vi "Euler sieve.vi"() -> ()   [LabVIEW 2021]
uses:
  <vilib>/Utility/file.llb/Write Delimited Spreadsheet (I64).vi
panel:
  in  "Path":path
  out "Running Time":dbl
  out "Array 2":u64[](array[numeric])
  out "Array":bool[](array[boolean])
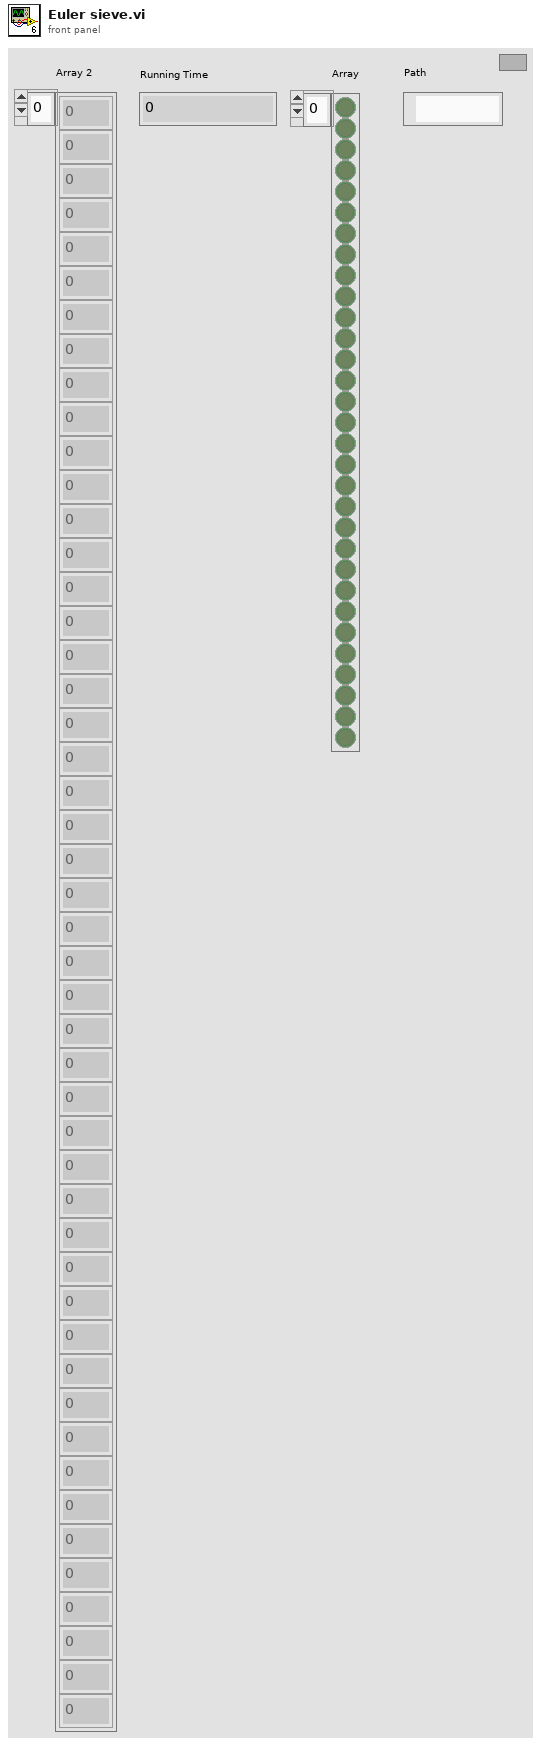
[diagram p1: front panel]
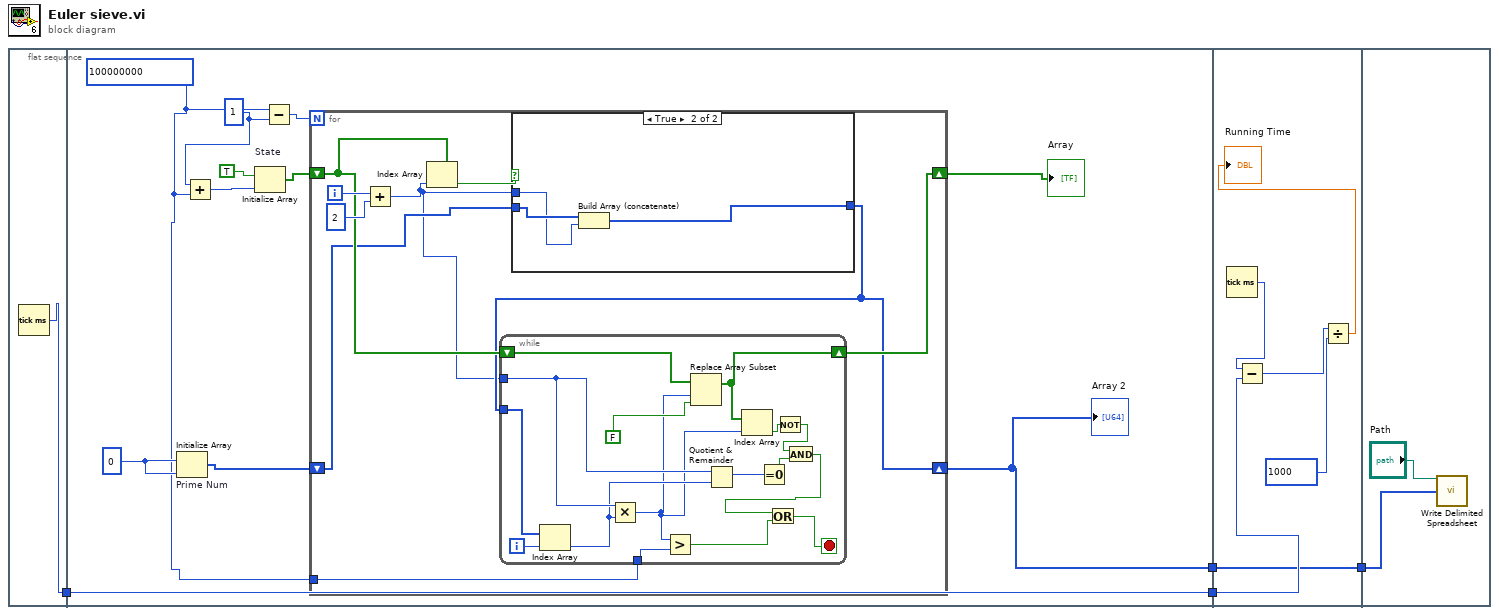
[diagram p0: block diagram]
diagram:
  n1 = flat-sequence {
    tunnel: [w5] -> w3
    tunnel: [w7] -> w4
    tunnel: w3 -> [w7]
    tunnel: [w6] -> w1
    tunnel: w4 -> [w50]
    tunnel: [w46] -> w2
    tunnel: w1 -> [w46]
    tunnel: w2 -> [w53]
    frame #0 {
      n2 = Tick Count (ms)() -> (millisecond timer value=w5:u32)
    }
    frame #1 {
      w12 = 0
      w15 = 1
      w9 = 100000000
      n3 = Initialize Array "Prime Num"(w12, w12) -> (w10:i32[])
      n4 = Add(x=w15, y=w9) -> (x+y=w14:i32)
      n5 = Initialize Array "State"(TRUE, w14) -> (w11:bool[])
      n6 = Subtract(x=w9, y=w15) -> (x-y=w16:i32)
      n7 = for {
        N: w16 -> [_]
        shift-right: [w21] -> w8
        shift-left: w11 -> [w20]
        shift-right: [w19] -> w6
        shift-left: w10 -> [w18]
        tunnel: w9 -> [w22]
        i -> [w25]
        n8 = Add(x=w25, y=2) -> (x+y=w17:i32)
        n9 = Index Array(array=w20, index=w17) -> (element=w23:bool)
        n10 = case shown="True" w23 {
          tunnel: w18 -> [w42 w44]
          tunnel: [w42 w45] -> w19
          tunnel: w17 -> [_ w43]
          frame False {
          }
          frame True {
            n11 = Build Array (concatenate)(w44, w43) -> (w45:i32[])
          }
        }
        n12 = while {
          tunnel: w17 -> [w38]
          tunnel: w22 -> [w39]
          shift-right: [w33] -> w21
          shift-left: w20 -> [w35]
          tunnel: w19 -> [w41]
          i -> [w40]
          stop <- w26 stop-if-true
          n13 = Index Array(array=w41, index=w40) -> (element=w37:i32)
          n14 = Multiply(x=w38, y=w37) -> (x*y=w32:i32)
          n15 = Greater?(x=w32, y=w39) -> (0:w28:bool)
          n16 = Replace Array Subset(array=w35, new element=FALSE, index=w32) -> (w33:bool[])
          n17 = Quotient & Remainder(x=w38, y=w37) -> (x-y*floor(x/y)=w34:i32)  [unwired: 1 out]
          n18 = Index Array(array=w33, index=w32) -> (element=w29:bool)
          n19 = Equal To 0?(x=w34) -> (x = 0?=w31:bool)
          n20 = Not(x=w29) -> (.not. x?=w30:bool)
          n21 = And(x=w30, y=w31) -> (x .and. y?=w27:bool)
          n22 = Or(x=w27, y=w28) -> (x .or. y?=w26:bool)
        }
      }
      "Array 2" <- w6
      "Array" <- w8
    }
    frame #2 {
      n23 = Tick Count (ms)() -> (millisecond timer value=w51:u32)
      n24 = Subtract(x=w51, y=w50) -> (x-y=w48:u32)
      n25 = Divide(x=w48, y=1000) -> (x/y=→"Running Time":dbl)
    }
    frame #3 {
      n26 = call-poly <vilib>:"Write Delimited Spreadsheet.vi"("file path (dialog if empty)"="Path", "1D data"=w53) -> ()  [unwired: 12 in, 2 out]
    }
  }
